vi "Notify Observers (State) Varient Input.vi"(7 "Expand Clusters":bool, 8 "error in (no error)":errorcluster, 9 "Data":variant, 10 "Label (default=taken from Data wire)":string, 11 "ObserverRegistry in":refnum<class "ObserverRegistry.lvclass">) -> (0 "error out":errorcluster, 3 "ObserverRegistry out":refnum<class "ObserverRegistry.lvclass">)   [LabVIEW 2011, in "Messenging.lvlib" / "ObserverRegistry.lvclass"]
uses:
  ObserverRegistry.lvclass
  Interprocess Messenger/TextVarientMessage/MSG.lvclass
  Interprocess Messenger/TextVarientMessage/Write VarMessage.vi
  Interprocess Messenger/VarMessage/VarMessage.lvclass
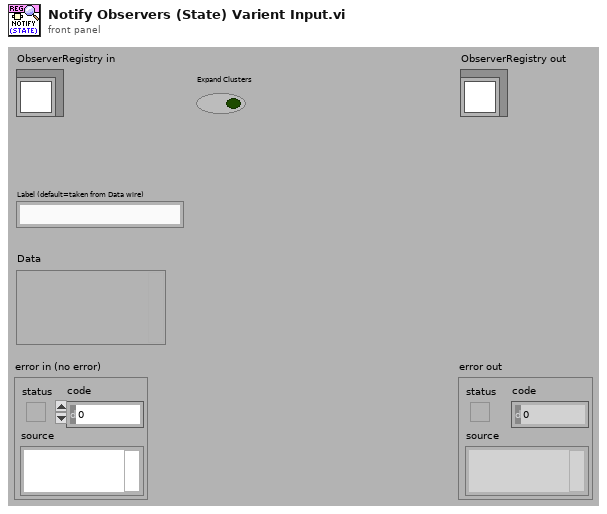
[diagram p1: front panel]
types:
  T1 = typedef "Type Descriptor Enumeration__ogtk.ctl" = enum8{"<Null>", "I8", "I16", "I32", "I64", "U8", "U16", "U32", "U64", "SGL", "DBL", "EXT", "CSG", "CDB", "CXT", "0x0F", "0x10", "0x11", "0x12", "0x13", "0x14", "Enum U8", "Enum U16", "Enum U32", "Enum U64", "SGL PQ", "DBL PQ", "EXT PQ", "CSG PQ", "CDB PQ", "CXT PQ", "0x1F", "0x20", "Boolean", "0x22", "0x23", "0x24", "0x25", "0x26", "0x27", "0x28", "0x29", "0x2A", "0x2B", "0x2C", "0x2D", "0x2E", "0x2F", "String", "0x31", "Path", "Pict", "0x34", "0x35", "0x36", "DAQ", "0x38", "0x39", "0x3A", "0x3B", "0x3C", "0x3D", "0x3E", "0x3F", "Array", "0x41", "0x42", "0x43", "0x44", "0x45", "0x46", "0x47", "0x48", "0x49", "0x4A", "0x4B", "0x4C", "0x4D", "0x4E", "0x4F", "Cluster", "0x51", "0x52", "Variant", "Waveform", "0x55", "0x56", "0x57", "0x58", "0x59", "0x5A", "0x5B", "0x5C", "0x5D", "0x5E", "0x5F", "0x60", "0x61", "0x62", "0x63", "0x64", "0x65", "0x66", "0x67", "0x68", "0x69", "0x6A", "0x6B", "0x6C", "0x6D", "0x6E", "0x6F", "Refnum"}
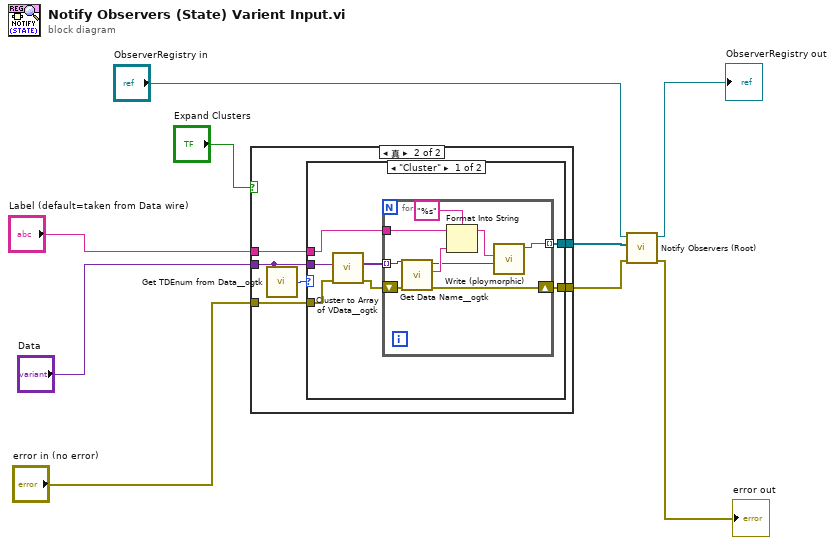
[diagram p0: block diagram]
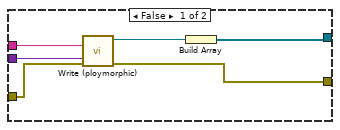
[diagram p2: hidden frame]
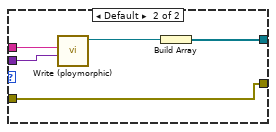
[diagram p3: hidden frame]
diagram:
  n1 = case shown="真" "Expand Clusters" {
    tunnel: "Label (default=taken from Data wire)" -> [w14 w21]
    tunnel: [w10 w20] -> w5
    tunnel: "Data" -> [w13 w19]
    tunnel: "error in (no error)" -> [w12 w17]
    tunnel: [w11 w16] -> w2
    frame False {
      n2 = call-poly "Write (ploymorphic).vi"("error in (no error)"=w12, "Varient"=w13, "Label"=w14) -> ("error out"=w11:errorcluster, "Message"=w15:refnum<class "VarMessage.lvclass">)  [unwired: 7 out]
      n3 = Build Array(w15) -> (w10:refnum<class "VarMessage.lvclass">[])
    }
    frame True {
      n4 = call <userlib>:"Get TDEnum from Data__ogtk.vi"("Data"=w19) -> ("Type Descriptor Enumeration"=w18:T1)  [unwired: 4 out]
      n5 = case shown="\"Cluster\"" w18 {
        tunnel: w21 -> [w26 w42]
        tunnel: [w25 w38] -> w20
        tunnel: w19 -> [w28 w40]
        tunnel: w17 -> [w24 w39]
        tunnel: [w22 w39] -> w16
        frame "Cluster" {
          n6 = call <userlib>:"Cluster to Array of VData__ogtk.vi"("error in (no error)"=w24, "Cluster"=w28) -> ("error out"=w23:errorcluster, "Array of VData"=w27:variant[])  [unwired: 8 out]
          n7 = for {
            tunnel: w27 -> [w37] mode=indexing
            tunnel: w26 -> [w35]
            tunnel: [w31] -> w25 mode=indexing
            shift-right: [w29] -> w22
            shift-left: w23 -> [w30]
            n8 = call <userlib>:"Get Data Name__ogtk.vi"("error in (no error)"=w30, "Data"=w37) -> ("error out"=w29:errorcluster, "Data Name"=w34:string, "Data dup"=w32:variant)  [unwired: 7 out]
            n9 = Format Into String(format string="%s", initial string=w35, w34) -> (resulting string=w33:string)  [unwired: 1 in, 1 out]
            n10 = call-poly "Write (ploymorphic).vi"("Varient"=w32, "Label"=w33) -> ("Message"=w31:refnum<class "VarMessage.lvclass">)  [unwired: 1 in, 8 out]
          }
        }
        frame Default {
          n11 = call-poly "Write (ploymorphic).vi"("Varient"=w40, "Label"=w42) -> ("Message"=w41:refnum<class "VarMessage.lvclass">)  [unwired: 1 in, 8 out]
          n12 = Build Array(w41) -> (w38:refnum<class "VarMessage.lvclass">[])
        }
      }
    }
  }
  n13 = call "Notify Observers (Root).vi"("error in (no error)"=w2, "Array of State Messages"=w5, "ObserverRegistry in"="ObserverRegistry in") -> ("error out"=→"error out":errorcluster, "ObserverRegistry out"=→"ObserverRegistry out":refnum<class "ObserverRegistry.lvclass">)  [unwired: 1 in, 6 out]
